vi "Destroy.vi"(8 "error in (no error)":errorcluster, 11 "CIF_NIChn_Fifo_Power_DVR in":refnum<class "CIF_NIChn_Fifo_Power_DVR.lvclass">) -> (0 "error out":errorcluster, 3 "CIF_NIChn_Fifo_Power_DVR out":refnum<class "CIF_NIChn_Fifo_Power_DVR.lvclass">)   [LabVIEW 2021, in "CIF_NIChn_Fifo_Power_DVR.lvclass"]
uses:
  CIF_NIChn_Fifo_Power_DVR.lvclass
  D:/dev/Packages/Channel_Manager/src/CIF_NIChn/NIChn/CIF_NIChn.lvclass
  D:/dev/Packages/Channel_Manager/src/CIFChannels/CIFChannels.lvclass
  NIChn/CIF_NIChn.lvclass/CIF_NIChn.ctl
  CIFChannels/CIFChannels.lvclass/CIFChannels.ctl
  CIF_NIChn_Fifo_Power_DVR.lvclass/CIF_NIChn_Fifo_Power_DVR.ctl
  ChannelCommon/typedef/Datatype Waveform.ctl
  <vilib>/CIF Foundation/CIF Channels/CIFChannels/SubVIs/CIFServices Fill In Error Info Ex.vi
  <vilib>/CIF Foundation/CIF Channels/CIFChannels/SubVIs/Get dll Path.vi
  <vilib>/CIF Foundation/CIF Utilities/Errors/Append Error Location.vi
  <vilib>/CIF Foundation/CIF Channels/CIFChannels/CIFChannelCore.lvlib
  NIChn/CIF_NIChn.lvclass
  CIFChannels/CIFChannels.lvclass
  ChannelCommon/ChannelCommon.lvlib
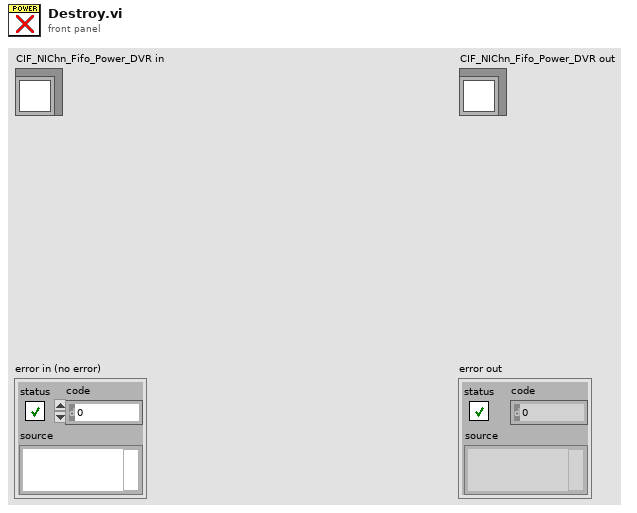
[diagram p1: front panel]
types:
  T1 = typedef "CIFChannels.lvclass/Direction.ctl" = enum16{"Publisher", "Subscriber"}
  T2 = typedef "ChannelCommon.lvlib/Datatype Waveform.ctl" = cluster{"measurement":dbl[], "dT":dbl, "Timestamp":i64, "Read Lock":bool}
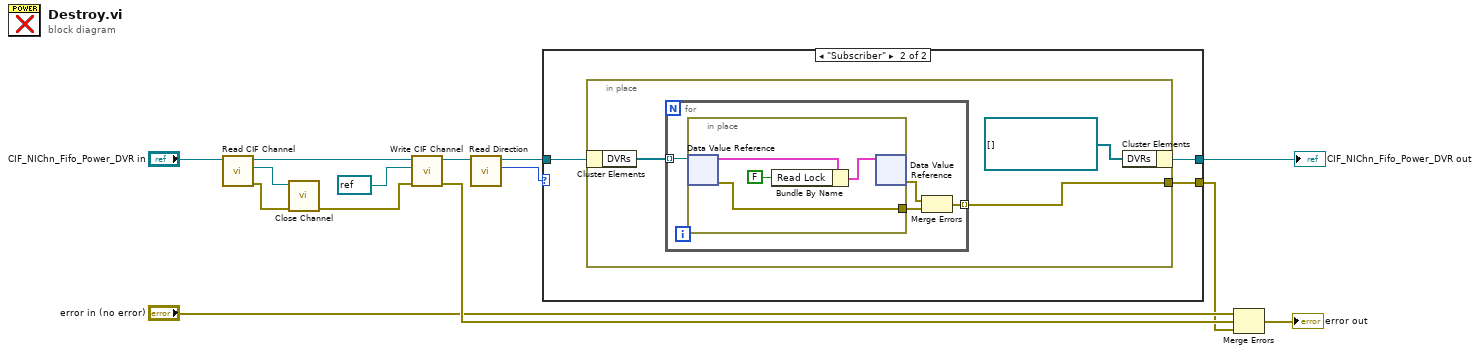
[diagram p0: block diagram]
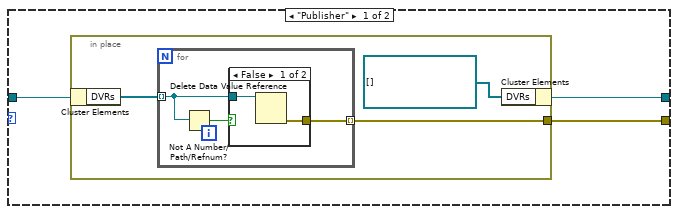
[diagram p2: hidden frame]
diagram:
  n1 = call "Read CIF Channel.vi"("CIFTag in"="CIF_NIChn_Fifo_Power_DVR in") -> ("error out"=w8:errorcluster, "CIF Channel"=w12:refnum<k21>, "CIFTag out"=w10:refnum<class "CIF_NIChn_Fifo_Power_DVR.lvclass">)  [unwired: 8 in]
  n2 = call <vilib>:"Close Channel.vi"("error in"=w8, "CIF Channel"=w12) -> ("error out"=w9:errorcluster)  [unwired: 9 in]
  n3 = call "Write CIF Channel.vi"("error in (no error)"=w9, "CIF Channel"=refnum<k21> refnum, "CIFTag in"=w10) -> ("error out"=w4:errorcluster, "CIFTag out"=w7:refnum<class "CIF_NIChn_Fifo_Power_DVR.lvclass">)  [unwired: 7 in]
  n4 = call "Read Direction.vi"("CIFChannels in"=w7) -> ("Direction"=w6:T1, "CIFChannels out"=w5:refnum<class "CIF_NIChn_Fifo_Power_DVR.lvclass">)  [unwired: 8 in, 1 out]
  n5 = case shown="\"Subscriber\"" w6 {
    tunnel: [w17 w28] -> w14
    tunnel: w5 -> [w16 w27]
    tunnel: [w15 w26] -> w2
    frame "Publisher" {
      n6 = in-place {
        in-place-border: [w18] -> w15
        n7 = in-place-cluster #1(w16) -> ("DVRs"=w20:refnum<data-value>[])
        n8 = for {
          tunnel: w20 -> [w22] mode=indexing
          tunnel: [w23] -> w18 mode=indexing
          n9 = Not A Number/Path/Refnum?(number/path/refnum=w22) -> (NaN/Path/Refnum?=w21:bool)
          n10 = case shown="False" w21 {
            tunnel: [w25 _] -> w23
            tunnel: w22 -> [w24 _]
            frame False {
              n11 = Delete Data Value Reference(data value reference=w24) -> (error out=w25:errorcluster)  [unwired: 1 in, 1 out]
            }
            frame True {
            }
          }
        }
        n12 = in-place-cluster #1("DVRs"=refnum<data-value>[] []) -> (w17:refnum<class "CIF_NIChn_Fifo_Power_DVR.lvclass">)
      }
    }
    frame "Subscriber" {
      n13 = in-place {
        in-place-border: [w29] -> w26
        n14 = in-place-cluster #2(w27) -> ("DVRs"=w30:refnum<data-value>[])
        n15 = for {
          tunnel: w30 -> [w35] mode=indexing
          tunnel: [w32] -> w29 mode=indexing
          n16 = in-place {
            in-place-border: [w39] -> w34
            n17 = in-place-dvr #3(w35) -> (w38:T2, w39:errorcluster)
            n18 = Bundle By Name(cluster=w38, "Read Lock"=FALSE) -> (w37:T2)
            n19 = in-place-dvr #3(w37) -> (w33:errorcluster)  [unwired: 1 out]
          }
          n20 = Merge Errors(w33, w34) -> (w32:errorcluster)
        }
        n21 = in-place-cluster #2("DVRs"=refnum<data-value>[] []) -> (w28:refnum<class "CIF_NIChn_Fifo_Power_DVR.lvclass">)
      }
    }
  }
  "CIF_NIChn_Fifo_Power_DVR out" <- w14
  n22 = Merge Errors("error in (no error)", w4, w2) -> (→"error out":errorcluster)
